vi "Close SMO.vi"(8 "error in (no error)":errorcluster, 11 "Instrument in":refnum<class "Instrument.lvclass">) -> (0 "error out":errorcluster, 3 "Instrument out":refnum<class "Instrument.lvclass">)   [LabVIEW 2019, in "Instrument.lvclass"]
uses:
  Instrument.lvclass
  Instrument.lvclass/Instrument.ctl
  <userlib>/LevyLab/RemoteControl/RemoteControl/RemoteControl.lvclass
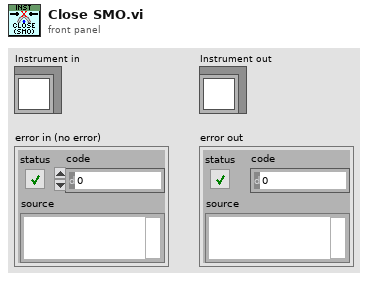
[diagram p1: front panel]
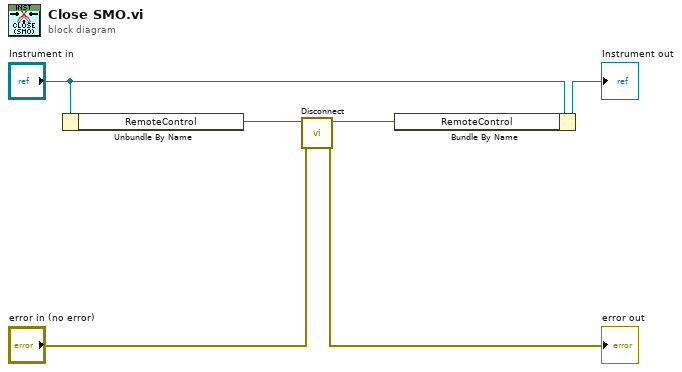
[diagram p0: block diagram]
diagram:
  n1 = Unbundle By Name("Instrument in") -> ("RemoteControl"=w2:refnum<class "RemoteControl.lvclass">)
  n2 = call <userlib>:"Disconnect.vi"("error in (no error)"="error in (no error)", "RemoteControl in"=w2) -> ("error out"=→"error out":errorcluster, "RemoteControl out"=w4:refnum<class "RemoteControl.lvclass">)  [unwired: 8 in]
  n3 = Bundle By Name(cluster="Instrument in", "RemoteControl"=w4) -> (→"Instrument out":refnum<class "Instrument.lvclass">)
